vi "Demo_Num to Bool.vi"(10 "PLC_Data":T1, 11 "Meassage IN":T2) -> (1 "Input Array":bool[](array[boolean]), 2 "Output Array":bool[](array[boolean]), 3 "Inputs":bool[](array[boolean]))   [LabVIEW 2017]
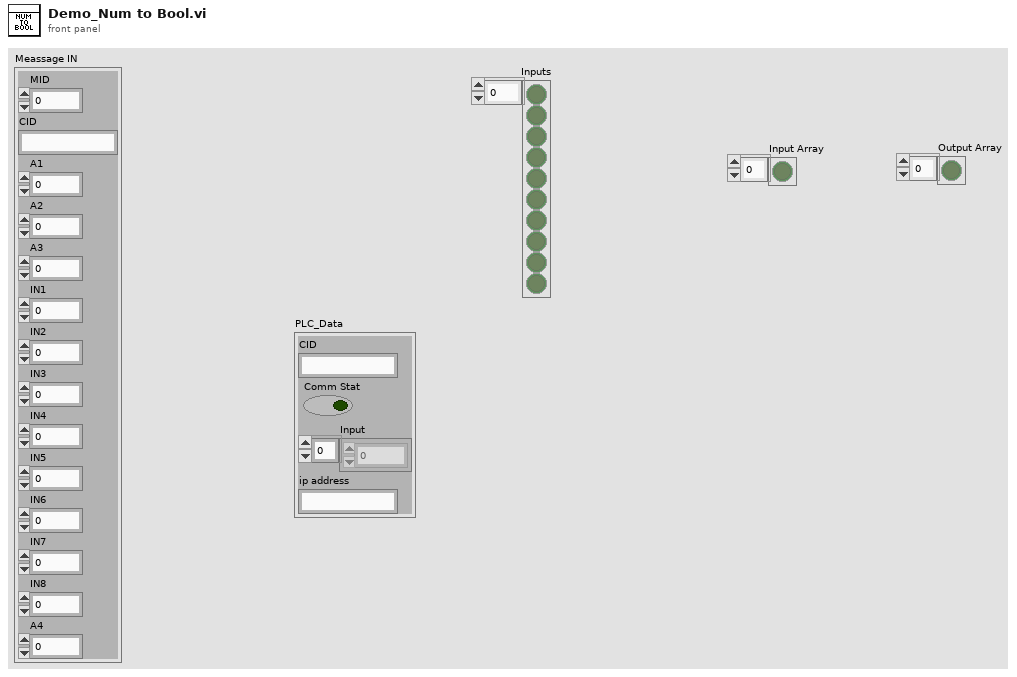
[diagram p1: front panel]
types:
  T1 = cluster{"CID":string, "Comm Stat":bool, "Input":u16[], "ip address":string}
  T2 = cluster{"MID":dbl, "CID":string, "A1":dbl, "A2":dbl, "A3":dbl, "IN1":u8, "IN2":u8, "IN3":u8, "IN4":u8, "IN5":u8, "IN6":u8, "IN7":u8, "IN8":u8, "A4":dbl}
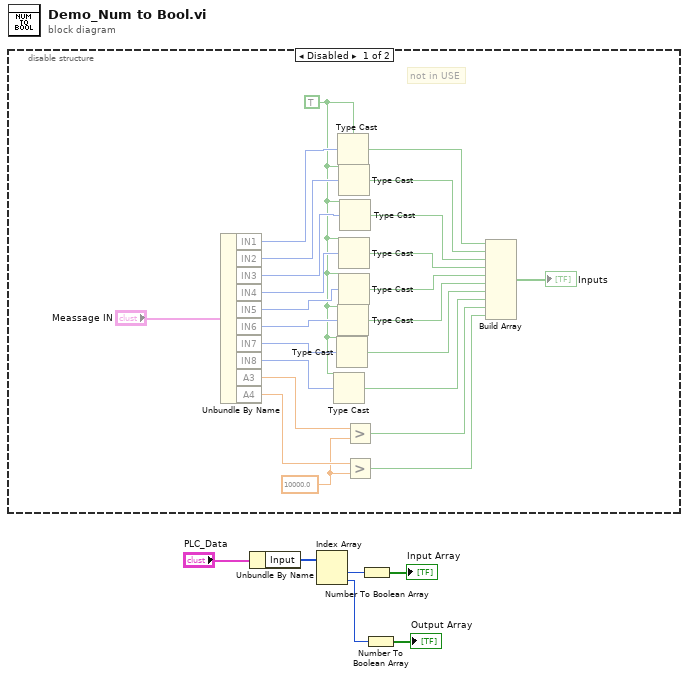
[diagram p0: block diagram]
diagram:
  n1 = disable-structure shown="Disabled" {
    frame Disabled {
      w9 = 10000.0 ("y")
      w22 = TRUE
      # "not in USE"
      n2 = Unbundle By Name("Meassage IN") -> ("IN1"=w23:u8, "IN2"=w24:u8, "IN3"=w25:u8, "IN4"=w26:u8, "IN5"=w27:u8, "IN6"=w28:u8, "IN7"=w29:u8, "IN8"=w30:u8, "A3"=w11:dbl, "A4"=w10:dbl)
      n3 = Type Cast(type=w22, x=w30) -> (*(type *) &x=w13:bool)
      n4 = Type Cast(type=w22, x=w29) -> (*(type *) &x=w14:bool)
      n5 = Type Cast(type=w22, x=w23) -> (*(type *) &x=w20:bool)
      n6 = Type Cast(type=w22, x=w28) -> (*(type *) &x=w15:bool)
      n7 = Type Cast(type=w22, x=w24) -> (*(type *) &x=w19:bool)
      n8 = Type Cast(type=w22, x=w26) -> (*(type *) &x=w17:bool)
      n9 = Type Cast(type=w22, x=w27) -> (*(type *) &x=w16:bool)
      n10 = Type Cast(type=w22, x=w25) -> (*(type *) &x=w18:bool)
      n11 = Greater?(x=w11, y=w9) -> (0:w8:bool)
      n12 = Greater?(x=w10, y=w9) -> (0:w7:bool)
      n13 = Build Array(w20, w19, w18, w17, w16, w15, w14, w13, w8, w7) -> (→"Inputs":bool[])
    }
    frame Enabled {
    }
  }
  n14 = Unbundle By Name("PLC_Data") -> ("Input"=w5:u16[])
  n15 = Index Array(array=w5) -> (element #1=w4:u16, element #2=w3:u16)  [unwired: 2 in]
  n16 = Number To Boolean Array(number=w4) -> (Boolean array=→"Input Array":bool[])
  n17 = Number To Boolean Array(number=w3) -> (Boolean array=→"Output Array":bool[])
